vi "Read Read Only.vi"(8 "error in (no error)":errorcluster, 11 "Const_Bool in":refnum<class "Const_Bool.lvclass">) -> (0 "error out":errorcluster, 2 "Read Only":bool, 3 "Const_Bool out":refnum<class "Const_Bool.lvclass">)   [LabVIEW 2021, in "Const_Bool.lvclass"]
uses:
  Const_Bool.lvclass
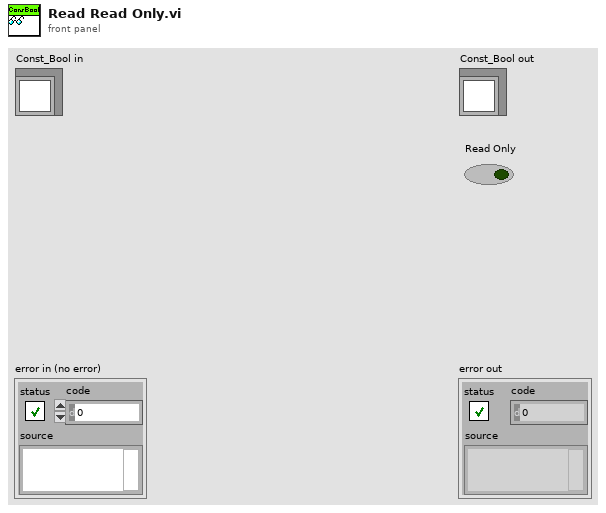
[diagram p1: front panel]
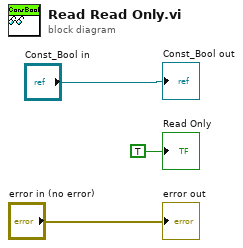
[diagram p0: block diagram]
diagram:
  "error out" <- "error in (no error)"
  "Const_Bool out" <- "Const_Bool in"
  "Read Only" <- TRUE ("Read Only")
